vi "list concentration to array.vi"(6 "Type":enum16{"List to Array", "Array to List"}(ring), 10 "List String In":string[][](array[string]), 11 "List Concentration In":T1(array[cluster]) {"N. Peak" items=["0.000000", "1.000000", "2.000000", "3.000000", "4.000000", "5.000000", "6.000000", "7.000000", "8.000000", "9.000000", "10.000000", "11.000000", "12.000000", "13.000000", "14.000000", "15.000000", "16.000000", "17.000000", "18.000000", "19.000000", "20.000000", "21.000000", "22.000000", "23.000000", "24.000000", "25.000000", "26.000000", "27.000000", "28.000000"]}) -> (2 "List Concentration Out":T1(array[cluster]) {"N. Peak" items=["0.000000", "1.000000", "2.000000", "3.000000", "4.000000", "5.000000", "6.000000", "7.000000", "8.000000", "9.000000", "10.000000", "11.000000", "12.000000", "13.000000", "14.000000", "15.000000", "16.000000", "17.000000", "18.000000", "19.000000", "20.000000", "21.000000", "22.000000", "23.000000", "24.000000", "25.000000", "26.000000", "27.000000", "28.000000"]}, 3 "List String Out":string[][](array[string]))   [LabVIEW 2023]
panel:
  in  "conc":T2 {"N. Peak" items=["1"=1, "2"=2, "3"=3, "4"=4]}
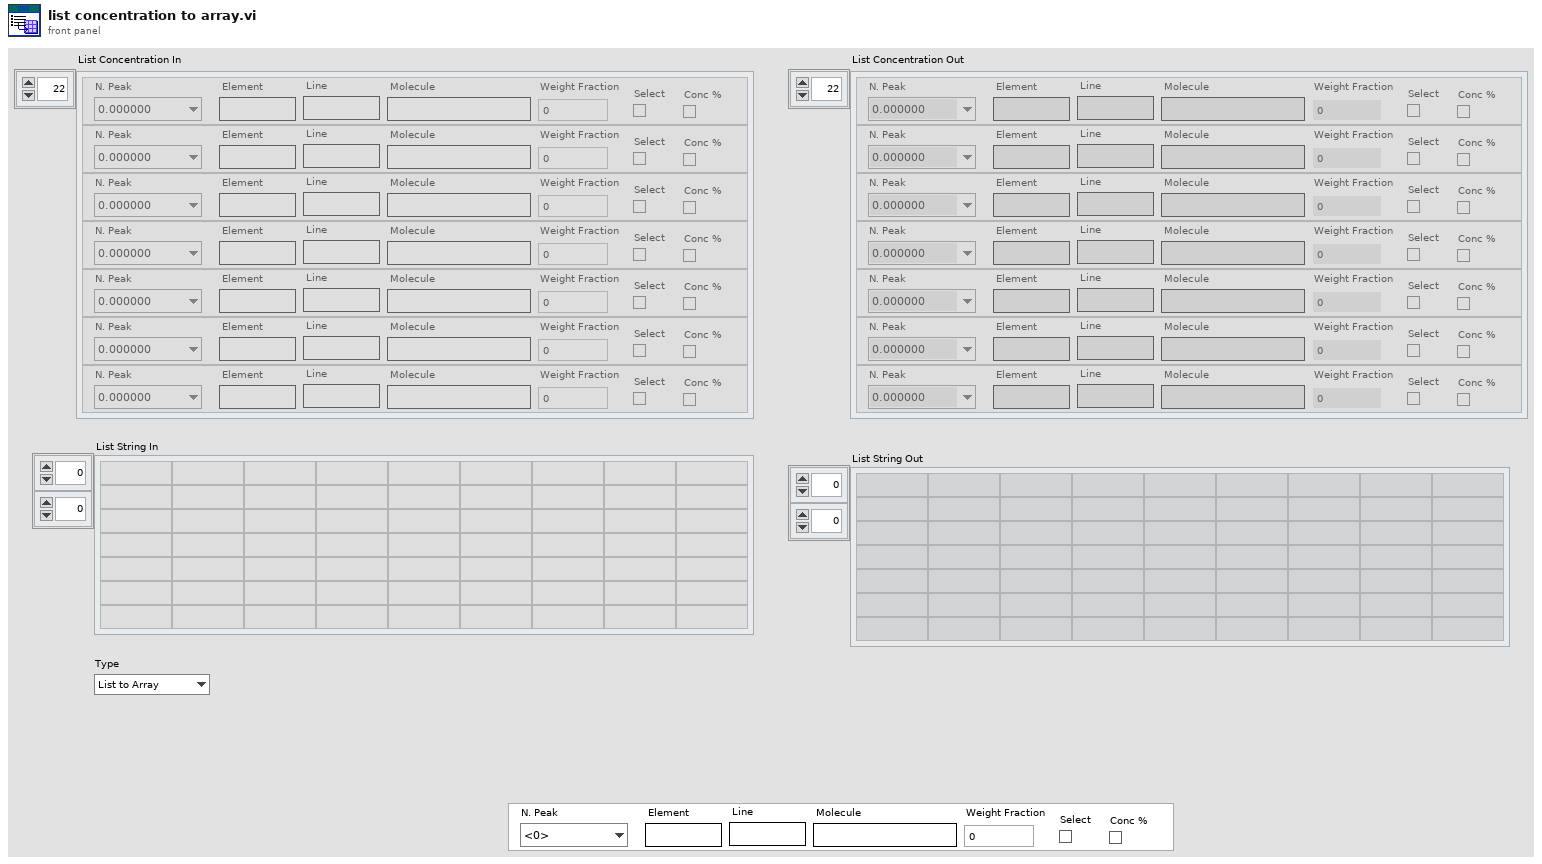
[diagram p1: front panel]
types:
  T1 = cluster{"N. Peak":u16, "Element":string, "Molecule":string, "Weight Fraction":dbl, "Select":bool, "Conc %":bool, "Line":string}[]
  T2 = cluster{"N. Peak":u16, "Element":string, "Molecule":string, "Weight Fraction":dbl, "Select":bool, "Conc %":bool, "Line":string}
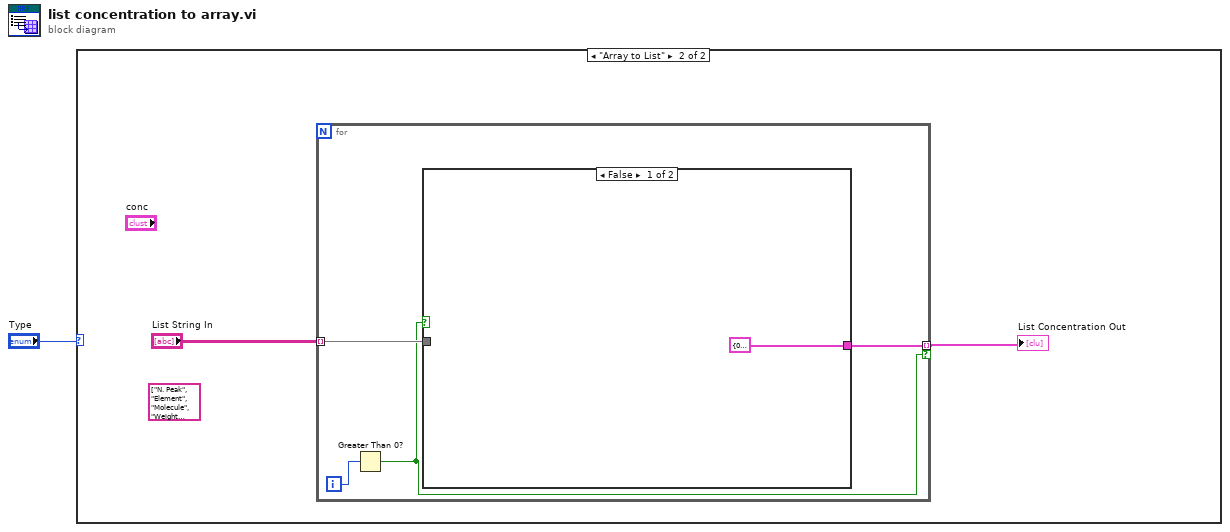
[diagram p0: block diagram]
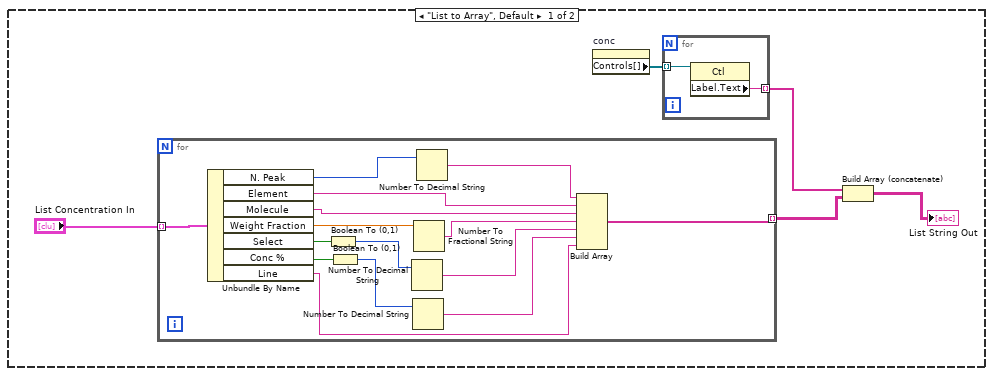
[diagram p2: hidden frame]
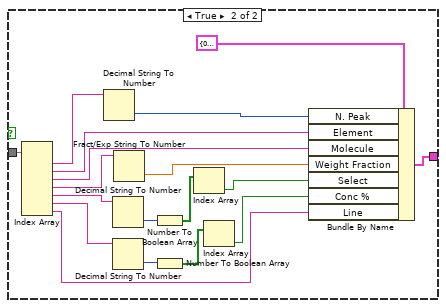
[diagram p3: hidden frame]
diagram:
  n1 = case shown="\"Array to List\"" "Type" {
    frame "List to Array", Default {
      n2 = for {
        tunnel: "List Concentration In" -> [w23] mode=indexing
        tunnel: [w11] -> w4 mode=indexing
        n3 = Unbundle By Name(w23) -> ("N. Peak"=w22:u16, "Element"=w15:string, "Molecule"=w10:string, "Weight Fraction"=w21:dbl, "Select"=w20:bool, "Conc %"=w19:bool, "Line"=w9:string)
        n4 = Boolean To (0,1)(Boolean=w20) -> (0, 1=w18:i16)
        n5 = Boolean To (0,1)(Boolean=w19) -> (0, 1=w17:i16)
        n6 = Number To Decimal String(number=w18) -> (decimal integer string=w13:string)  [unwired: 1 in]
        n7 = Number To Decimal String(number=w17) -> (decimal integer string=w12:string)  [unwired: 1 in]
        n8 = Number To Fractional String(number=w21) -> (F-format string=w14:string)  [unwired: 3 in]
        n9 = Number To Decimal String(number=w22) -> (decimal integer string=w16:string)  [unwired: 1 in]
        n10 = Build Array(w16, w15, w10, w14, w13, w12, w9) -> (w11:string[])
      }
      n11 = property on="conc" class="Clust (strict)"() -> ("Controls[]"=w6:refnum<vi>[])  [unwired: 2 in, 2 out]
      n12 = for {
        tunnel: w6 -> [w8] mode=indexing
        tunnel: [w7] -> w5 mode=indexing
        n13 = property class="Ctl"(reference=w8) -> ("Label.Text"=w7:string)  [unwired: 1 in, 2 out]
      }
      n14 = Build Array (concatenate)(w5, w4) -> (→"List String Out":string[][])
    }
    frame "Array to List" {
      (unwired) string[][] [["N. Peak", "Element", "Molecule", "Weight Fraction", "Select", "Conc %"], ["1", "", "", "0.000000", "0", "0"], ["2", "", "", "0.000000", "0", "0"]] ("List String Out")
      n15 = for {
        tunnel: [w29] -> w24 mode=indexing if=w26
        tunnel: "List String In" -> [w28] mode=indexing
        i -> [w27]
        n16 = Greater Than 0?(x=w27) -> (x > 0?=w26:bool)
        n17 = case shown="False" w26 {
          tunnel: [T2 {"N. Peak"=0, "Element"="", "Molecule"="", "Weight Fraction"=0.0, "Select"=FALSE, "Conc %"=FALSE, "Line"=""} ("conc") w48] -> w29
          tunnel: w28 -> [_ w47]
          frame False {
          }
          frame True {
            n18 = Index Array(array=w47) -> (element #1=w46:string, element #2=w44:string, element #3=w43:string, element #4=w42:string, element #5=w40:string, element #6=w39:string, element #7=w31:string)  [unwired: 7 in]
            n19 = Decimal String To Number(string=w46) -> (number=w45:i32)  [unwired: 2 in, 1 out]
            n20 = Decimal String To Number(string=w40) -> (number=w38:i32)  [unwired: 2 in, 1 out]
            n21 = Decimal String To Number(string=w39) -> (number=w37:i32)  [unwired: 2 in, 1 out]
            n22 = Fract/Exp String To Number(string=w42) -> (number=w41:dbl)  [unwired: 3 in, 1 out]
            n23 = Number To Boolean Array(number=w38) -> (Boolean array=w36:bool[])
            n24 = Number To Boolean Array(number=w37) -> (Boolean array=w34:bool[])
            n25 = Index Array(array=w36) -> (element=w35:bool)  [unwired: 1 in]
            n26 = Index Array(array=w34) -> (element=w33:bool)  [unwired: 1 in]
            n27 = Bundle By Name(cluster=T2 {"N. Peak"=0, "Element"="", "Molecule"="", "Weight Fraction"=0.0, "Select"=FALSE, "Conc %"=FALSE, "Line"=""} ("conc"), "N. Peak"=w45, "Element"=w44, "Molecule"=w43, "Weight Fraction"=w41, "Select"=w35, "Conc %"=w33, "Line"=w31) -> (w48:T2)
          }
        }
      }
      "List Concentration Out" <- w24
    }
  }
